vi "PlugIn PWM.vi"(6 "String Value":string, 10 "Channel":T2, 11 "Menu":T1=enum."get") -> ()   [LabVIEW 2019]
uses:
  <vilib>/Rock Robotics/SystemInterfaces/DIO/FPGA_DIOPWMChannel.ctl
  PWM Update Ops.ctl
panel:
  # "Don't place this VI anywhere\nin your API code. It needs to\nbe a dynamically loaded\nwrapper of the main global"
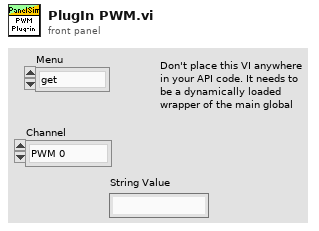
[diagram p1: front panel]
types:
  T1 = typedef "PWM Update Ops.ctl" = enum16{"set init", "set speed", "set position", "set raw", "set  period_scale", "set zero_latch", "set angular range", "get", "delete", "JSON update", "set name", "transmit initial", "reset"}
  T2 = typedef "FPGA_DIOPWMChannel.ctl" = enum8{"PWM 0", "PWM 1", "PWM 2", "PWM 3", "PWM 4", "PWM 5", "PWM 6", "PWM 7", "PWM 8", "PWM 9", "PWM MXP 0", "PWM MXP 1", "PWM MXP 2", "PWM MXP 3", "PWM MXP 4", "PWM MXP 5", "PWM MXP 6", "PWM MXP 7", "PWM MXP 8", "PWM MXP 9", "Invalid"}
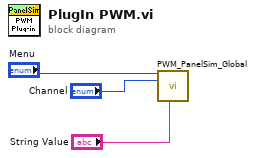
[diagram p0: block diagram]
diagram:
  n1 = call "PWM_PanelSim_Global.vi"("menu"="Menu", "PWMChannel"="Channel", "String Value"="String Value") -> ()  [unwired: 11 in, 2 out]
